vi "DDS9959 Set CFR.vi"(2 "error in (no error)":errorcluster, 3 "Channel":u16=4 min=1 max=4, 4 "Channel Function Register":T1={"0=cos, 1=sin"=FALSE, "clear phase accum"=FALSE, "autoclear phase accum"=FALSE, "clear sweep accum"=FALSE, "autoclear sweep accum"=FALSE, "match pipe delays"=FALSE, "DAC power down"=FALSE, "digital power down"=FALSE, "DAC current (8)"=TRUE, "DAC current (9)"=TRUE, "Must be 0"=FALSE, "Open"=FALSE, "Open"=FALSE, "Sweep ramp rate timer"=FALSE, "Sweep enable"=FALSE, "Sweep no-dwell"=FALSE, "Open"=FALSE, "Open"=FALSE, "Open"=FALSE, "Open"=FALSE, "Open"=FALSE, "Open 2"=FALSE, "AFP mod select (22)"=FALSE, "AFP mod select (23)"=FALSE}, 5 "VISA resource name":refnum<visa-resource-name>="USB0::0x0456::0xEE07::NI-VISA-0::RAW") -> (0 "error out":errorcluster, 1 "VISA resource name out":refnum<visa-resource-name>="USB0::0x0456::0xEE07::NI-VISA-0::RAW")   [LabVIEW 2012]
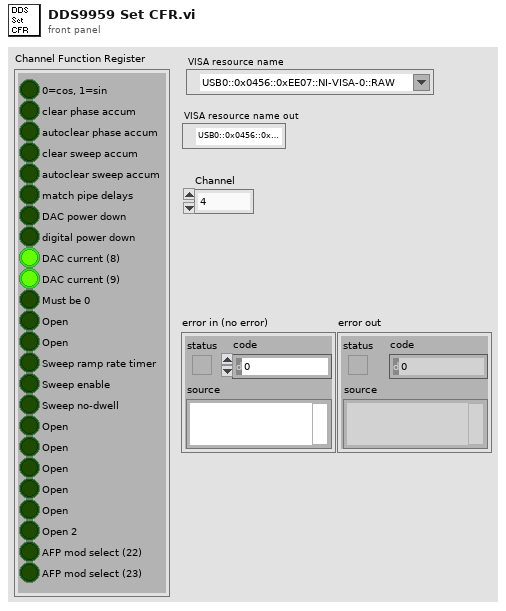
[diagram p1: front panel]
types:
  T1 = cluster{"0=cos, 1=sin":bool, "clear phase accum":bool, "autoclear phase accum":bool, "clear sweep accum":bool, "autoclear sweep accum":bool, "match pipe delays":bool, "DAC power down":bool, "digital power down":bool, "DAC current (8)":bool, "DAC current (9)":bool, "Must be 0":bool, "Open":bool, "Open":bool, "Sweep ramp rate timer":bool, "Sweep enable":bool, "Sweep no-dwell":bool, "Open":bool, "Open":bool, "Open":bool, "Open":bool, "Open":bool, "Open 2":bool, "AFP mod select (22)":bool, "AFP mod select (23)":bool}
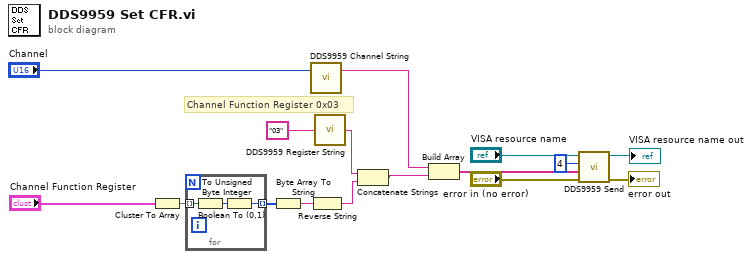
[diagram p0: block diagram]
diagram:
  # "Channel Function Register 0x03"
  n1 = Cluster To Array(cluster="Channel Function Register") -> (array=w4:bool[])
  n2 = for {
    tunnel: w4 -> [w17] mode=indexing
    tunnel: [w18] -> w7 mode=indexing
    n3 = Boolean To (0,1)(Boolean=w17) -> (0, 1=w19:i16)
    n4 = To Unsigned Byte Integer(number=w19) -> (unsigned 8bit integer=w18:u8)
  }
  n5 = Byte Array To String(unsigned byte array=w7) -> (string=w6:string)
  n6 = call "DDS9959 Channel String.vi"("Channel"="Channel") -> ("String"=w2:string)  [unwired: 2 in]
  n7 = Reverse String(1:w6) -> (0:w5:string)
  n8 = call "DDS9959 Register String.vi"("register"="03") -> ("output"=w11:string)
  n9 = Concatenate Strings(w11, w5) -> (w10:string)
  n10 = Build Array(w2, w10) -> (w16:string[])
  n11 = call "DDS9959 Send.vi"("error in (no error)"="error in (no error)", "Output Array"=w16, "USB Out Endpoint"=i16 4, "VISA resource name"="VISA resource name") -> ("error out"=→"error out":errorcluster, "VISA resource name"=→"VISA resource name out":refnum<visa-resource-name>)  [unwired: 6 in]
